vi "Self Test.vi"(8 "error in":errorcluster, 11 "4300 in":refnum<class "4300.lvclass">) -> (0 "error out":errorcluster, 3 "4300 out":refnum<class "4300.lvclass">)   [LabVIEW 2019, in "4300.lvlib" / "4300.lvclass"]
doc: "This VI should implement the device specific method for self test used to verify the device is connected and operational with no faults present. If a fault is present, return a boolean. The connect override is the only VI that should call this VI and should throw an error if the self test fails."
uses:
  Library/4300.lvclass
  builds/Instruments/AnalogInput.lvlibp/Library/AnalogInput.lvclass
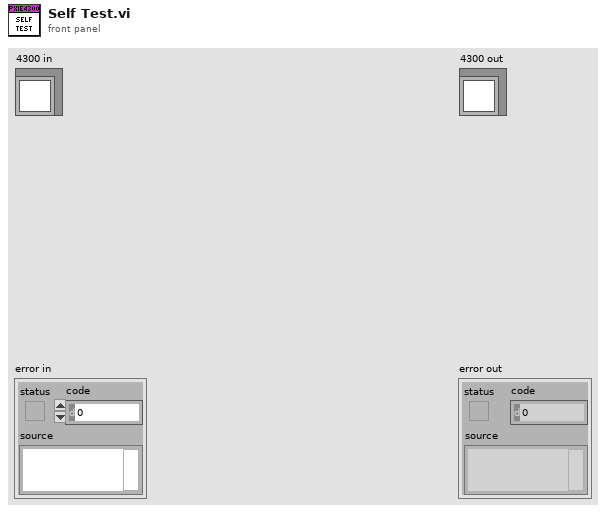
[diagram p1: front panel]
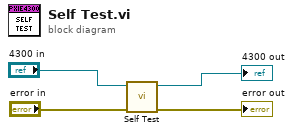
[diagram p0: block diagram]
diagram:
  n1 = call-parent "Self Test.vi"("error in"="error in", "Instruments in"="4300 in") -> ("error out"=→"error out":errorcluster, "Instruments out"=→"4300 out":refnum<class "4300.lvclass">)  [unwired: 8 in]
